vi "getDeviceType.vi"(8 "error in (no error)":errorcluster, 11 "DigitalDevice.lvclass in":refnum<class "DigitalDevice.lvclass">) -> (0 "error out":errorcluster, 2 "type":T1(ring), 3 "DigitalDevice.lvclass out":refnum<class "DigitalDevice.lvclass">)   [LabVIEW 2011, in "Tools.lvlib" / "DatabaseHelpers.lvlib" / "DigitalDevice.lvclass"]
uses:
  DigitalDevice.lvclass
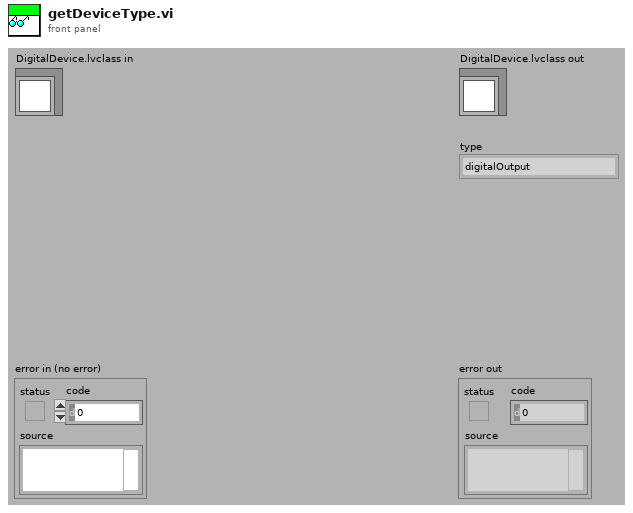
[diagram p1: front panel]
types:
  T1 = enum16{"digitalOutput", "digitalInput", "analogOutput", "analogInput", "rfOutput", "ethernetSupply"}
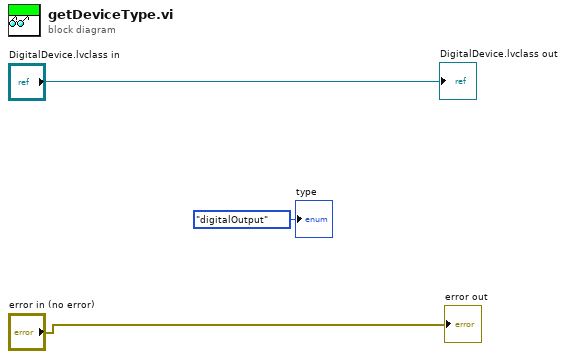
[diagram p0: block diagram]
diagram:
  "error out" <- "error in (no error)"
  "DigitalDevice.lvclass out" <- "DigitalDevice.lvclass in"
  "type" <- T1."digitalOutput" ("type")
